vi "solar_voy Write (Relay).vi"(6 "Suppress Errors? (T)":bool=TRUE, 7 "TARGET":string, 8 "error in (no error)":errorcluster, 9 "Variant (No HDR)":variant, 10 "PACKET":string, 11 "Voyager Refnum in":T1) -> (0 "error out":errorcluster, 3 "Voyager Refnum out":T1)   [LabVIEW 2018]
doc: "This relays a local command back to COSMOS using the 'HANDSHAKE' packet. If the packet is not registered, this does nothing. The 'HANDSHAKE' packet sets the 'ORIGIN' == LCL."
uses:
  solar_voy_def/solar_voy_def_ctl HANDSHAKE.ctl
  solar_voy_ctl Voyager Refnum.ctl
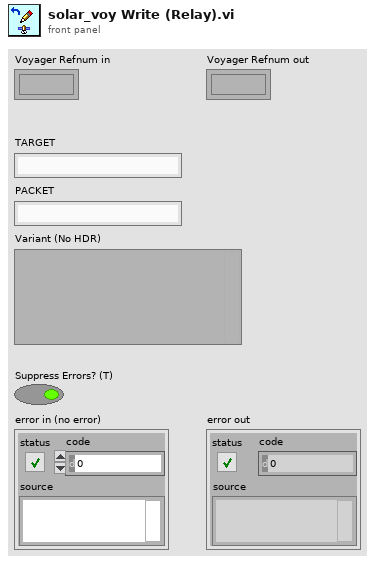
[diagram p1: front panel]
types:
  T1 = typedef "solar_voy_ctl Voyager Refnum.ctl" = refnum<k1>
  T2 = typedef "solar_voy_def_ctl HANDSHAKE.ctl" = cluster{"ORIGIN":enum8{"RMT", "LCL"}, "STATUS,s=OK,ERROR":bool, "CODE":i32, "TIME_SECONDS":u32, "TIME_MICROSECONDS":u32, "DATA,t=BLOCK":string}
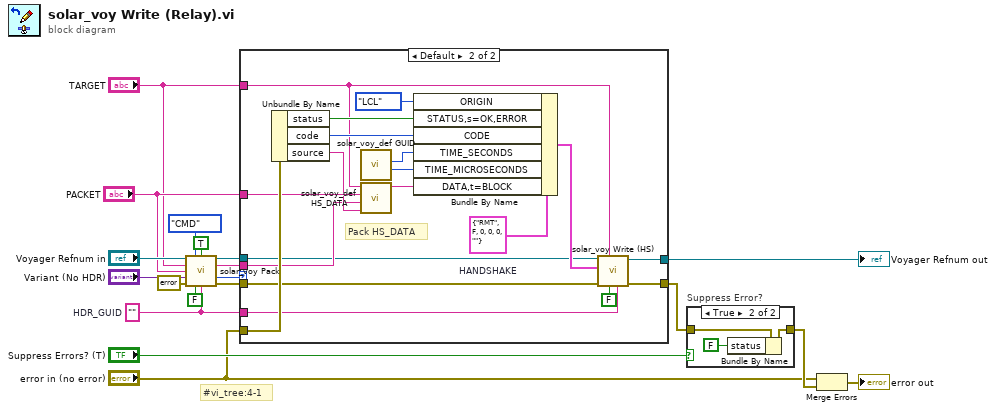
[diagram p0: block diagram]
diagram:
  w4 = ""  # HDR_GUID
  # "#vi_tree:4-1"
  n1 = call "solar_voy Pack.vi"("Voyager Refnum in"="Voyager Refnum in", "CMD"=enum8{"CMD", "TLM"}."CMD", "Update Last Value? (F)"=TRUE, "TARGET"="TARGET", "PACKET (\"\" = Use Variant)"="PACKET", "Variant (No HDR)"="Variant (No HDR)", "error in (no error)"=errorcluster {"status"=FALSE, "code"=0, "source"=""}, "Suppress Errors? (T)"=FALSE, "HDR_GUID"=w4) -> ("Voyager Refnum out"=w12:T1, "TCP Data to Send"=w5:string, "Packet Index"=w7:i32, "error out"=w6:errorcluster)  [unwired: 3 in]
  n2 = case shown="Default" w7 {
    tunnel: [w20 w40] -> w16
    tunnel: [w21 w39] -> w15
    tunnel: "error in (no error)" -> [_ w34]
    tunnel: w12 -> [w21 w22]
    tunnel: "TARGET" -> [_ w28]
    tunnel: "PACKET" -> [_ w27]
    tunnel: w6 -> [w20 w23]
    tunnel: w5 -> [_ w24]
    tunnel: w4 -> [_ w25]
    frame -1 {
      # "CMD PACKET not defined\n- Do nothing"
    }
    frame Default {
      w37 = T2 {"ORIGIN"=enum."RMT", "STATUS,s=OK,ERROR"=FALSE, "CODE"=0, "TIME_SECONDS"=0, "TIME_MICROSECONDS"=0, "DATA,t=BLOCK"=""}  # HANDSHAKE
      # "Pack HS_DATA"
      n3 = Unbundle By Name(w34) -> ("status"=w33:bool, "code"=w32:i32, "source"=w26:string)
      n4 = call "solar_voy_def GUID.vi"() -> ("TIME_MICROSECONDS"=w30:u32, "TIME_SECONDS"=w31:u32)  [unwired: 8 in, 2 out]
      n5 = call "solar_voy_def HS_DATA.vi"("Error Source"=w26, "PACKET_DATA"=w24, "PACKET"=w27, "TARGET"=w28) -> ("HS_DATA"=w29:string)  [unwired: 7 in]
      n6 = Bundle By Name(cluster=w37, "ORIGIN"=enum8{"RMT", "LCL"}."LCL", "STATUS,s=OK,ERROR"=w33, "CODE"=w32, "TIME_SECONDS"=w31, "TIME_MICROSECONDS"=w30, "DATA,t=BLOCK"=w29) -> (w36:T2)
      n7 = call "solar_voy Write (HS).vi"("HDR_GUID"=w25, "Suppress Errors? (T)"=FALSE, "TARGET"=w28, "error in (no error)"=w23, "HANDSHAKE"=w36, "Voyager Refnum in"=w22) -> ("error out"=w40:errorcluster, "Voyager Refnum out"=w39:T1)  [unwired: 4 in]
    }
  }
  "Voyager Refnum out" <- w15
  n8 = case "Suppress Error?" shown="True" "Suppress Errors? (T)" {
    tunnel: w16 -> [w41 w44]
    tunnel: [w41 w43] -> w18
    frame False {
    }
    frame True {
      n9 = Bundle By Name(cluster=w44, "status"=FALSE) -> (w43:errorcluster)
    }
  }
  n10 = Merge Errors("error in (no error)", w18) -> (→"error out":errorcluster)
